vi "generate galvo waveforms.vi"(8 "error in (no error)":errorcluster, 11 "Waveform in":refnum<class "Waveform.lvclass">) -> (0 "error out":errorcluster, 1 "Waveform 2":waveform(dbl), 2 "Waveform":waveform(dbl), 3 "Waveform out":refnum<class "Waveform.lvclass">)   [LabVIEW 2012, in "Waveform.lvclass"]
uses:
  Waveform.lvclass
  Waveform.lvclass/Waveform.ctl
panel:
  out "wfm2":waveform(dbl)(graph)
  out "wfm1":waveform(dbl)(graph)
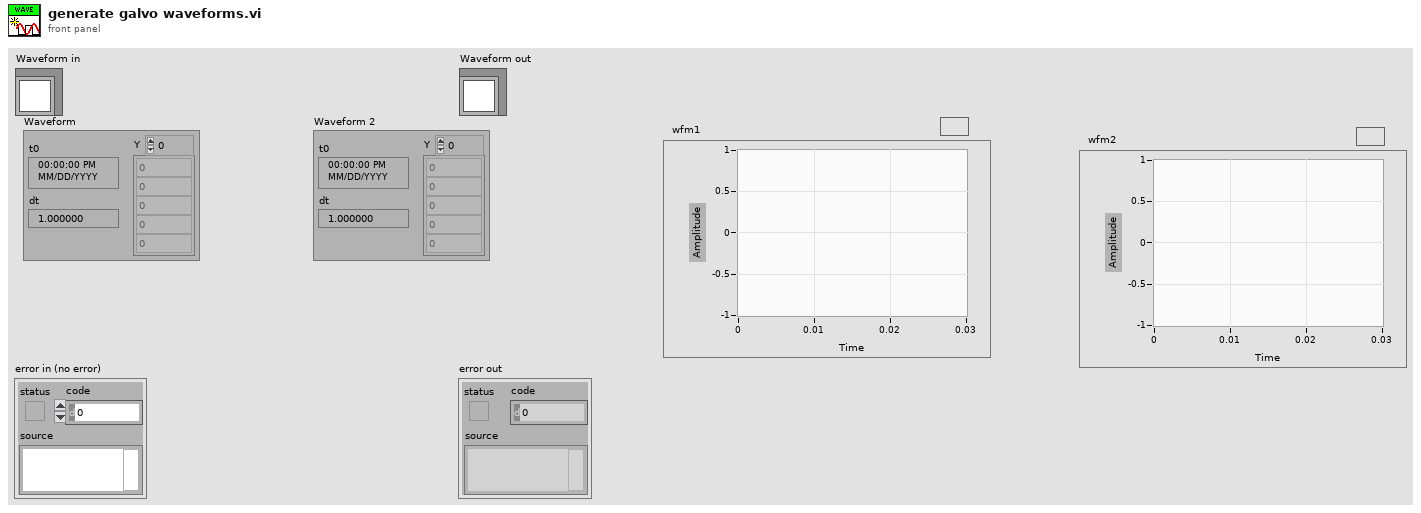
[diagram p1: front panel]
types:
  T1 = typedef "Waveform.lvclass/waveform data.ctl" = cluster{"amplitude":dbl[unit], "offset":dbl[unit], "delay":dbl[unit], "duty cycle":dbl, "sampling info":cluster{"Fs":dbl, "#s":dbl}, "frequency":dbl[unit], "phase":dbl[unit]}
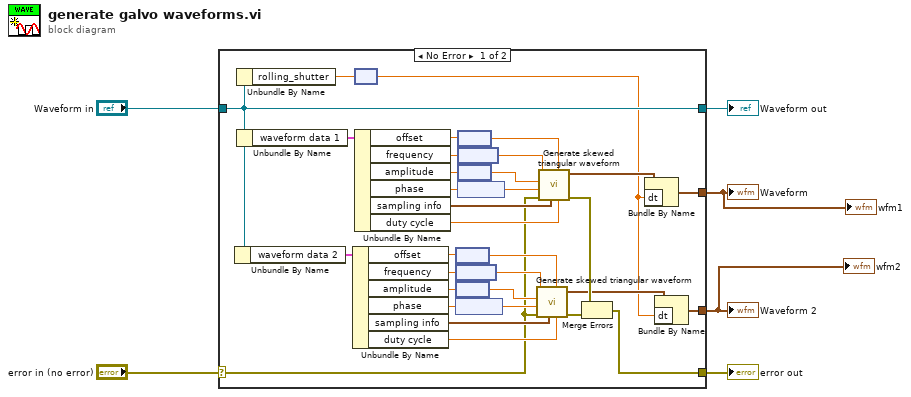
[diagram p0: block diagram]
diagram:
  n1 = case shown="No Error" "error in (no error)" {
    selector: "error in (no error)" -> [w15 w41]
    tunnel: [w14 w41] -> w5
    tunnel: [w13 w40] -> w3
    tunnel: "Waveform in" -> [w13 w40]
    tunnel: [w8 _] -> w2
    tunnel: [w7 _] -> w1
    frame No Error {
      n2 = Unbundle By Name(w13) -> ("waveform data 2"=w20:T1)
      n3 = Unbundle By Name(w13) -> ("rolling_shutter"=w12:dbl[unit])
      n4 = Unbundle By Name(w13) -> ("waveform data 1"=w39:T1)
      n5 = Unbundle By Name(w20) -> ("offset"=w22:dbl[unit], "frequency"=w23:dbl[unit], "amplitude"=w25:dbl[unit], "phase"=w27:dbl[unit], "sampling info"=w29:cluster{"Fs":dbl, "#s":dbl}, "duty cycle"=w18:dbl)
      n6 = node(w12) -> (w9:dbl)
      n7 = Unbundle By Name(w39) -> ("offset"=w37:dbl[unit], "frequency"=w36:dbl[unit], "amplitude"=w34:dbl[unit], "phase"=w32:dbl[unit], "sampling info"=w30:cluster{"Fs":dbl, "#s":dbl}, "duty cycle"=w19:dbl)
      n8 = node(w22) -> (w21:dbl)
      n9 = node(w23) -> (w24:dbl)
      n10 = node(w25) -> (w26:dbl)
      n11 = node(w27) -> (w28:dbl)
      n12 = node(w37) -> (w38:dbl)
      n13 = node(w36) -> (w35:dbl)
      n14 = node(w34) -> (w33:dbl)
      n15 = node(w32) -> (w31:dbl)
      n16 = call "Generate skewed triangular waveform.vi"("Duty cycle (%)"=w18, "Offset"=w21, "sampling info"=w29, "error in (no error)"=w15, "Phase"=w28, "Amplitude"=w26, "Frequency"=w24) -> ("error out"=w16:errorcluster, "Waveform"=w10:waveform(dbl))  [unwired: 3 in]
      n17 = call "Generate skewed triangular waveform.vi"("Duty cycle (%)"=w19, "Offset"=w38, "sampling info"=w30, "error in (no error)"=w15, "Phase"=w31, "Amplitude"=w33, "Frequency"=w35) -> ("error out"=w17:errorcluster, "Waveform"=w11:waveform(dbl))  [unwired: 3 in]
      n18 = Merge Errors(w17, w16) -> (w14:errorcluster)
      n19 = Bundle By Name(cluster=w11, "dt"=w9) -> (w8:waveform(dbl))
      n20 = Bundle By Name(cluster=w10, "dt"=w9) -> (w7:waveform(dbl))
    }
    frame Error {
    }
  }
  "error out" <- w5
  "Waveform out" <- w3
  "Waveform" <- w2
  "Waveform 2" <- w1
  "wfm1" <- w2
  "wfm2" <- w1
